vi "GetProcessRef.vi"(8 "error in (no error)":errorcluster, 11 "Edit in":refnum<class "Edit.lvclass">) -> (0 "error out":errorcluster, 2 "Static VI Ref":refnum<vi>, 3 "Edit out":refnum<class "Edit.lvclass">)   [LabVIEW 2019, in "Edit.lvclass"]
uses:
  Edit.lvclass
  C:/Program Files (x86)/National Instruments/LabVIEW 2019/vi.lib/JKI/JKI SMO/SMO/SMO.lvclass
  <vilib>/JKI/JKI SMO/SMO/SMO.lvclass/SMO.ctl
  <vilib>/JKI/JKI SMO/SMO/Private/ReftoDVR--SMO.vi
  <vilib>/JKI/JKI SMO/SMO/SMO.lvclass
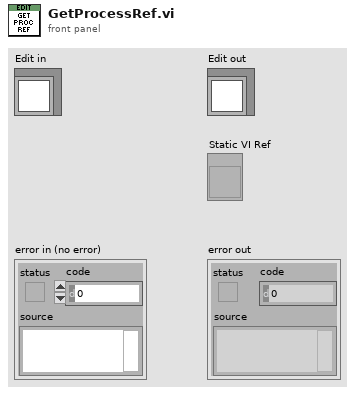
[diagram p1: front panel]
types:
  T1 = typedef "SMO.lvclass/RegisteredProcessData--Cluster.ctl" = cluster{"Name":string, "Static VI Ref":refnum<vi>, "Running":bool, "NotifierRef":u32}
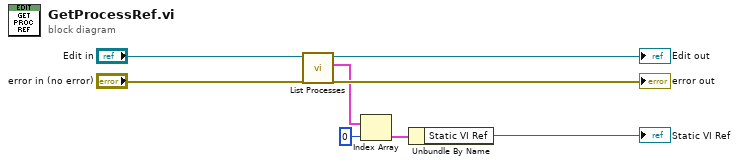
[diagram p0: block diagram]
diagram:
  n1 = call <vilib>:"List Processes.vi"("error in (no error)"="error in (no error)", "SMO"="Edit in") -> ("error out"=→"error out":errorcluster, "Registered Processes"=w3:T1[], "SMO out"=→"Edit out":refnum<class "Edit.lvclass">)  [unwired: 7 in]
  n2 = Index Array(array=w3, index=0) -> (element=w1:T1)
  n3 = Unbundle By Name(w1) -> ("Static VI Ref"=→"Static VI Ref":refnum<vi>)
